vi "Add Mapping.vi"(8 "error in (no error)":errorcluster, 11 "references":T1) -> (0 "error out":errorcluster, 3 "references out":T1)   [LabVIEW 2013, in "Scaling editor node.lvclass"]
uses:
  Scaling editor node.lvclass
  <vilib>/NI/DCAF Table API/Table Manager/object ref.ctl
  <vilib>/NI/Tag Bus Data Framework/Configuration Editor/Classes/Engine Parent/Engine Parent Editor Node.lvclass
  <vilib>/NI/Tag Bus Data Framework/Configuration Editor/Classes/Module editor node/module editor node.lvclass
  module/configuration/Scaling configuration.lvclass
  <vilib>/NI/DCAF Table API/Table Manager/Table Manager.lvclass
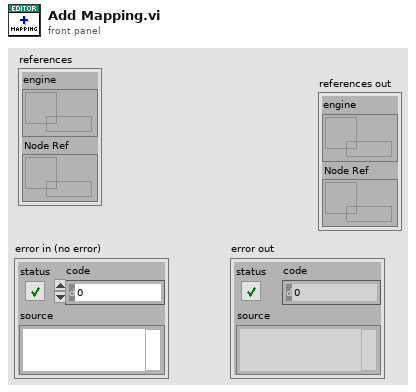
[diagram p1: front panel]
types:
  T1 = typedef "Table Manager.lvlib/Table Manager.lvclass/object ref.ctl" = cluster{"engine":refnum<data-value>, "Node Ref":refnum<data-value>}
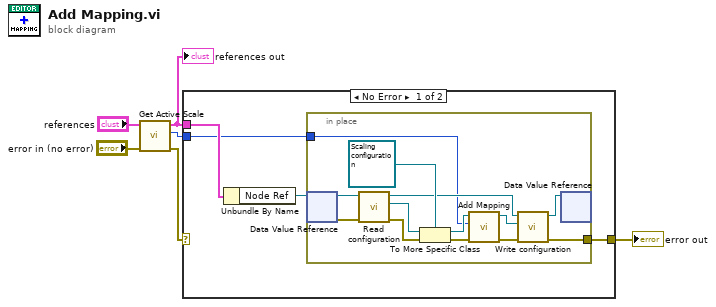
[diagram p0: block diagram]
diagram:
  n1 = call "Get Active Scale.vi"("error in (no error)"="error in (no error)", "references"="references") -> ("error out"=w2:errorcluster, "Index"=w1:i32, "references out"=w3:T1)  [unwired: 6 in]
  "references out" <- w3
  n2 = case shown="No Error" w2 {
    selector: w2 -> [_ w24]
    tunnel: [w10 w24] -> w6
    tunnel: w3 -> [w8 _]
    tunnel: w1 -> [w7 _]
    frame No Error {
      n3 = Unbundle By Name(w8) -> ("Node Ref"=w9:refnum<data-value>)
      n4 = in-place {
        in-place-border: [w16] -> w10
        in-place-border: w7 -> [w11]
        n5 = in-place-dvr #1(w9) -> (w14:refnum<class "module editor node.lvclass">, w23:errorcluster)
        n6 = call-dynamic "Read configuration.vi"("error in"=w23, "NISE_CEF_serializable node in"=w14) -> ("error out"=w20:errorcluster, "configuration"=w22:refnum<class "NISE_CEF_serializable configuration.lvclass">, "NISE_CEF_serializable node out"=w13:refnum<class "module editor node.lvclass">)  [unwired: 7 in]
        n7 = To More Specific Class(target class=refnum<class "Scaling configuration.lvclass"> refnum ("Scaling configuration"), reference=w22, error in=w20) -> (specific class reference=w19:refnum<class "Scaling configuration.lvclass">, error out=w18:errorcluster)
        n8 = call "Add Mapping.vi"("error in (no error)"=w18, "scale index"=w11, "Scaling configuration in"=w19) -> ("error out"=w15:errorcluster, "Scaling configuration out"=w17:refnum<class "Scaling configuration.lvclass">)  [unwired: 7 in]
        n9 = call-dynamic "Write configuration.vi"("error in"=w15, "configuration"=w17, "NISE_CEF_serializable node in"=w13) -> ("error out"=w16:errorcluster, "NISE_CEF_serializable node out"=w12:refnum<class "module editor node.lvclass">)  [unwired: 7 in]
        n10 = in-place-dvr #1(w12) -> ()  [unwired: 2 out]
      }
    }
    frame Error {
    }
  }
  "error out" <- w6
